vi "VariableIncreaseOverTime.vi"(5 "Reset to current":bool, 7 "Current value":dbl, 9 "Multiplier (units/sec)":dbl, 10 "Variable in":dbl, 11 "Joystick input":dbl) -> (2 "Variable out":dbl)   [LabVIEW 2014]
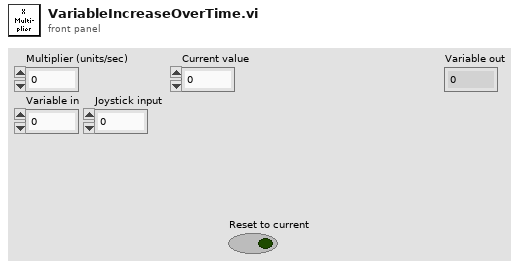
[diagram p1: front panel]
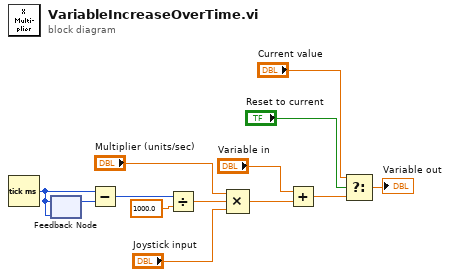
[diagram p0: block diagram]
diagram:
  n1 = Tick Count (ms)() -> (millisecond timer value=w12:u32)
  n2 = feedback #1(w12) -> (w13:u32)
  n3 = feedback-in #1(w12) -> ()
  n4 = Subtract(x=w12, y=w13) -> (x-y=w11:u32)
  n5 = Divide(x=w11, y=1000.0) -> (x/y=w9:dbl)
  n6 = Compound Arithmetic op=MULTIPLY("Multiplier (units/sec)", w9, "Joystick input") -> (w4:dbl)
  n7 = Add(x="Variable in", y=w4) -> (x+y=w6:dbl)
  n8 = Select(t="Current value", s="Reset to current", f=w6) -> (s? t:f=→"Variable out":dbl)
